vi "chart series set labels options.vi"(7 "show_value":u8, 8 "error in (no error)":errorcluster, 9 "show_category":u8, 10 "show_name":u8, 11 "series":u32) -> (0 "error out":errorcluster)   [LabVIEW 8.6]
doc: "void chart_series_set_labels_options(lxw_chart_series series, uint8_t show_name, uint8_t show_category, uint8_t show_value);"
uses:
  pending_lvxlsxwriter/xlsxwriter.dll
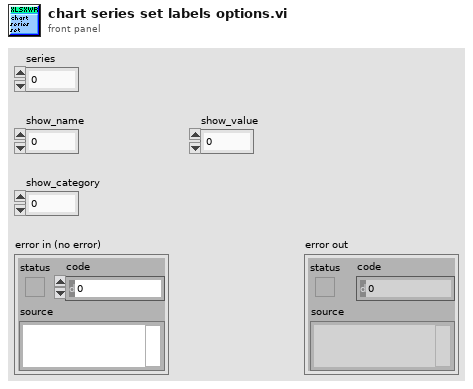
[diagram p1: front panel]
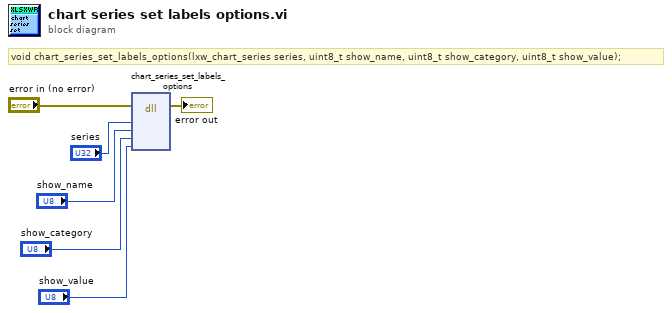
[diagram p0: block diagram]
diagram:
  # "void chart_series_set_labels_options(lxw_chart_series series, uint8_t show_name, uint8_t show_category, uint8_t show_value);"
  n1 = dll-call lib="C:/Users/WDAGUtilityAccount/Desktop/pending_lvxlsxwriter/xlsxwriter.*" fn="chart_series_set_labels_options"(error in="error in (no error)", "series"="series", "show_name"="show_name", "show_category"="show_category", "show_value"="show_value") -> (error out=→"error out":errorcluster)  [unwired: 7 in, 1 out]
